vi "Initialize Stop Process.vi"(8 "error in (no error)":errorcluster, 11 "Car Wash Model in":refnum<class "Car Wash Model.lvclass">) -> (0 "error out":errorcluster, 3 "Car Wash Model out":refnum<class "Car Wash Model.lvclass">)   [LabVIEW 2019, in "Car Wash Model.lvclass"]
uses:
  <vilib>/gpm_packages/@cs/Car-wash/Source/Car Wash Model/Car Wash Model/Car Wash Model.lvclass
  C:/Program Files/National Instruments/LabVIEW 2019/vi.lib/gpm_packages/@cs/mva-core/Source/IModel/IModel/IModel.lvclass
  <vilib>/gpm_packages/@cs/mva-core/Source/IObserver/IObserver/IObserver.lvclass/IObserver.ctl
  <vilib>/gpm_packages/@cs/mva-core/Source/IModel/IModel/IModel.lvclass/IModel.ctl
  <vilib>/gpm_packages/@cs/mva-core/Source/IMediator/PublishRequest/PublishRequest.lvclass/PublishRequest.ctl
  <vilib>/gpm_packages/@cs/mva-core/Source/IMediator/IMediator Messages/Publish Msg/Publish Msg.lvclass/Publish Msg.ctl
  <vilib>/gpm_packages/@cs/actor-framework-messages/Source/RoundTripMessage/RoundTripMessage.lvclass/RoundTripMessage.ctl
  <vilib>/ActorFramework/Message Enqueuer/Message Enqueuer.lvclass/Message Enqueuer.ctl
  <vilib>/gpm_packages/@cs/mva-core/Source/IMediator/IMediator Messages/Publish Msg/Send Pre-Addressed Publish.vi
  <vilib>/gpm_packages/@cs/mva-core/Source/IObserver/IObserver/Read Unique ID.vi
  <vilib>/gpm_packages/@cs/mva-core/Source/IMediator/PublishRequest/Pack Publish Request.vi
  <vilib>/gpm_packages/@cs/actor-framework-messages/Source/RoundTripMessage/Return Round-Trip Message.vi
  <vilib>/ActorFramework/Message Enqueuer/Enqueue.vi
  <vilib>/gpm_packages/@cs/mva-core/Source/IModel/IModel/IModel.lvclass
  C:/Program Files/National Instruments/LabVIEW 2019/vi.lib/gpm_packages/@cs/mva-core/Source/IObserver/IObserver/IObserver.lvclass
  <vilib>/gpm_packages/@cs/mva-core/Source/IMediator/IMediator Messages/Publish Msg/Publish Msg.lvclass
  C:/Program Files/National Instruments/LabVIEW 2019/vi.lib/gpm_packages/@cs/actor-framework-messages/Source/RoundTripMessage/RoundTripMessage.lvclass
  <vilib>/gpm_packages/@cs/actor-framework-messages/Source/RoundTripMessage/RoundTripMessage.lvclass
  C:/Program Files/National Instruments/LabVIEW 2019/vi.lib/ActorFramework/Message/Message.lvclass
  <vilib>/Utility/error.llb/Error Cluster From Error Code.vi
  <vilib>/ActorFramework/Message Priority Queue/Priority Enqueue.vi
  <vilib>/gpm_packages/@cs/mva-core/Source/IMediator/PublishRequest/PublishRequest.lvclass
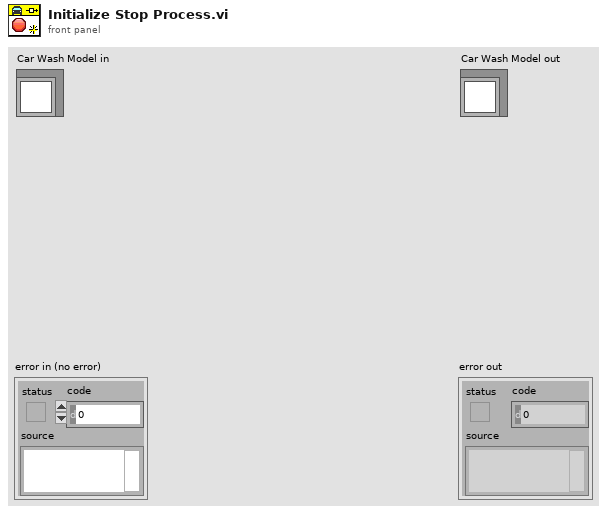
[diagram p1: front panel]
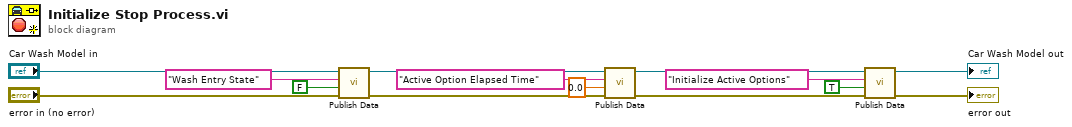
[diagram p0: block diagram]
diagram:
  n1 = call <vilib>:"Publish Data.vi"("error in (no error)"="error in (no error)", "Data to Publish"=FALSE, "Datum Name"="Wash Entry State" ("Datum Name (\"\"=Use Control Label)"), "IModel in"="Car Wash Model in") -> ("error out"=w9:errorcluster, "IModel out"=w10:refnum<class "Car Wash Model.lvclass">)  [unwired: 6 in]
  n2 = call <vilib>:"Publish Data.vi"("error in (no error)"=w9, "Data to Publish"=0.0, "Datum Name"="Active Option Elapsed Time" ("Datum Name (\"\"=Use Control Label)"), "IModel in"=w10) -> ("error out"=w4:errorcluster, "IModel out"=w6:refnum<class "Car Wash Model.lvclass">)  [unwired: 6 in]
  n3 = call <vilib>:"Publish Data.vi"("error in (no error)"=w4, "Data to Publish"=TRUE, "Datum Name"="Initialize Active Options", "IModel in"=w6) -> ("error out"=→"error out":errorcluster, "IModel out"=→"Car Wash Model out":refnum<class "Car Wash Model.lvclass">)  [unwired: 6 in]
